vi "Drive.vi"(7 "Slow?":bool, 9 "SwitchDir":bool=TRUE, 10 "Drive L":dbl, 11 "Drive R":dbl) -> ()   [LabVIEW 2016]
panel:
  in  "Drive Reduction":dbl=0.4 format="%#_13g"
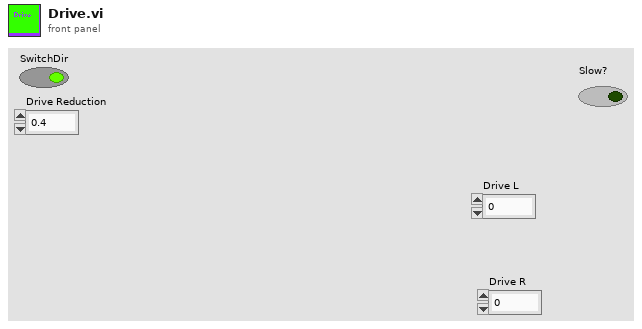
[diagram p1: front panel]
types:
  T1 = typedef "WPI_MotorControlDeviceRef.ctl" = cluster{"DeviceStatus":errorcluster, "Type":T2, "PWM":cluster{"PWM Channel":T3, "DeadBand":T4}, "CAN":cluster{"Device Number":u8, "SetOutput VI Ref":variant, "GetOutput VI Ref":variant, "Enable VI Ref":variant, "Disable VI Ref":variant, "Data":variant}, "Invert":bool}
  T2 = typedef "WPI_MotorControlType.ctl" = enum16{"PWM", "CAN"}
  T3 = typedef "FPGA_DIOPWMChannel.ctl" = enum8{"PWM 0", "PWM 1", "PWM 2", "PWM 3", "PWM 4", "PWM 5", "PWM 6", "PWM 7", "PWM 8", "PWM 9", "PWM MXP 0", "PWM MXP 1", "PWM MXP 2", "PWM MXP 3", "PWM MXP 4", "PWM MXP 5", "PWM MXP 6", "PWM MXP 7", "PWM MXP 8", "PWM MXP 9", "Invalid"}
  T4 = typedef "WPI_PWMDeadband.ctl" = cluster{"Name":string, "maxPositivePwm":i32, "minPositivePwm":i32, "centerPwm":i32, "maxNegativePwm":i32, "minNegativePwm":i32, "angularRange":u16}
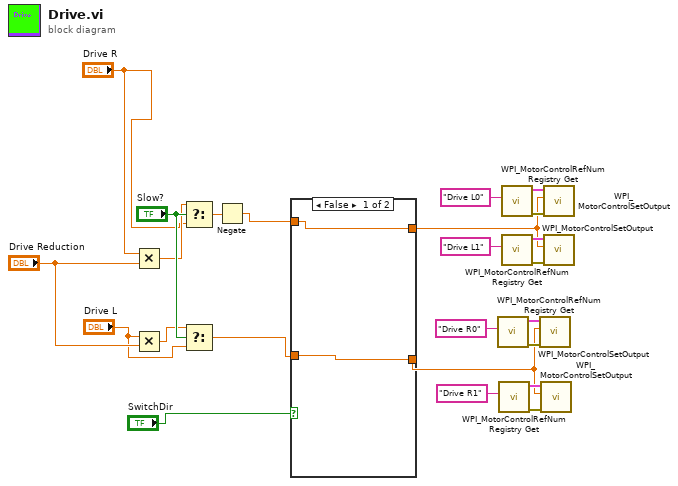
[diagram p0: block diagram]
diagram:
  n1 = Multiply(x="Drive R", y="Drive Reduction") -> (x*y=w4:dbl)
  n2 = Multiply(x="Drive L", y="Drive Reduction") -> (x*y=w2:dbl)
  n3 = Select(t=w4, s="Slow?", f="Drive R") -> (s? t:f=w11:dbl)
  n4 = Select(t=w2, s="Slow?", f="Drive L") -> (s? t:f=w7:dbl)
  n5 = Negate(x=w11) -> (-x=w9:dbl)
  n6 = case shown="False" "SwitchDir" {
    tunnel: [w26 w27] -> w10
    tunnel: w9 -> [w26 w28]
    tunnel: [w25 w28] -> w8
    tunnel: w7 -> [w25 w27]
    frame False {
    }
    frame True {
    }
  }
  n7 = call <vilib>:"WPI_MotorControlRefNum Registry Get.vi"("refnum name"="Drive R0") -> ("error out"=w18:errorcluster, "MotorControlDevRef"=w14:T1)  [unwired: 9 in]
  n8 = call <vilib>:"WPI_MotorControlRefNum Registry Get.vi"("refnum name"="Drive R1") -> ("error out"=w13:errorcluster, "MotorControlDevRef"=w16:T1)  [unwired: 9 in]
  n9 = call <vilib>:"WPI_MotorControlRefNum Registry Get.vi"("refnum name"="Drive L0") -> ("error out"=w19:errorcluster, "MotorControlDevRef"=w20:T1)  [unwired: 9 in]
  n10 = call <vilib>:"WPI_MotorControlRefNum Registry Get.vi"("refnum name"="Drive L1") -> ("error out"=w23:errorcluster, "MotorControlDevRef"=w22:T1)  [unwired: 9 in]
  n11 = call <vilib>:"WPI_MotorControlSetOutput.vi"("error in (no error)"=w18, "Output"=w8, "MotorControlDevRef"=w14) -> ()  [unwired: 6 in, 3 out]
  n12 = call <vilib>:"WPI_MotorControlSetOutput.vi"("error in (no error)"=w13, "Output"=w8, "MotorControlDevRef"=w16) -> ()  [unwired: 6 in, 3 out]
  n13 = call <vilib>:"WPI_MotorControlSetOutput.vi"("error in (no error)"=w19, "Output"=w10, "MotorControlDevRef"=w20) -> ()  [unwired: 6 in, 3 out]
  n14 = call <vilib>:"WPI_MotorControlSetOutput.vi"("error in (no error)"=w23, "Output"=w10, "MotorControlDevRef"=w22) -> ()  [unwired: 6 in, 3 out]
